vi "Msg.Q.Destroy.vi"(8 "Error (in)":errorcluster, 11 "Msg.Q.Ref":T1) -> (0 "Error (out)":errorcluster)   [LabVIEW 2023]
doc: "This VI is used to destroy a queue of message and data."
uses:
  Msg.Data.ctl
  Msg.Q.Ref.ctl
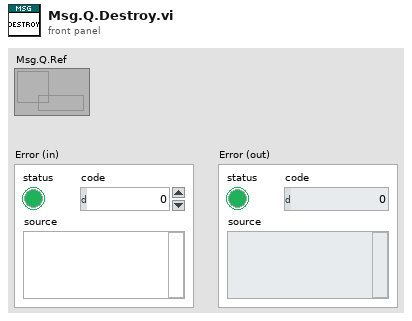
[diagram p1: front panel]
types:
  T1 = typedef "Msg.Q.Ref.ctl" = refnum<queue>
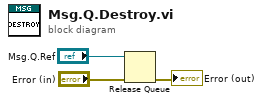
[diagram p0: block diagram]
diagram:
  n1 = Release Queue(queue="Msg.Q.Ref", error in (no error)="Error (in)") -> (error out=→"Error (out)":errorcluster)  [unwired: 1 in, 2 out]
